vi "KundtsTube2-week7J&J.vi"() -> ()   [LabVIEW 2015]
uses:
  <vilib>/Analysis/NI_AALPro.lvlib
  <vilib>/Analysis/2dsp.llb/Real FFT.vi
  <vilib>/express/express analysis/Spectral/XNode/ExpressSpectralMeasurementsBlockNode.xnode
  <vilib>/express/express analysis/Spectral/Block/exnSpectralBlock spectral measurements RMS poly.vi
  <vilib>/express/express analysis/Spectral/Block/exnSpectralBlock spectral measurements RMS WFM.vi
panel:
  out "?":cdb[](graph)
  out "FFT Graph":cdb[](graph)
  in  "stop":bool
  in  "Time (s)":dbl
  in  "Rate":dbl
  in  "Averages":dbl
  out "Results":T1
  out "Resonance Curve":cluster{"all rows":dbl[], "Array":dbl[]}[](graph)
  in  "Tab Control":enum32{"Simulation", "Experiment"}(tab)
  in  "Input Parameter":T2
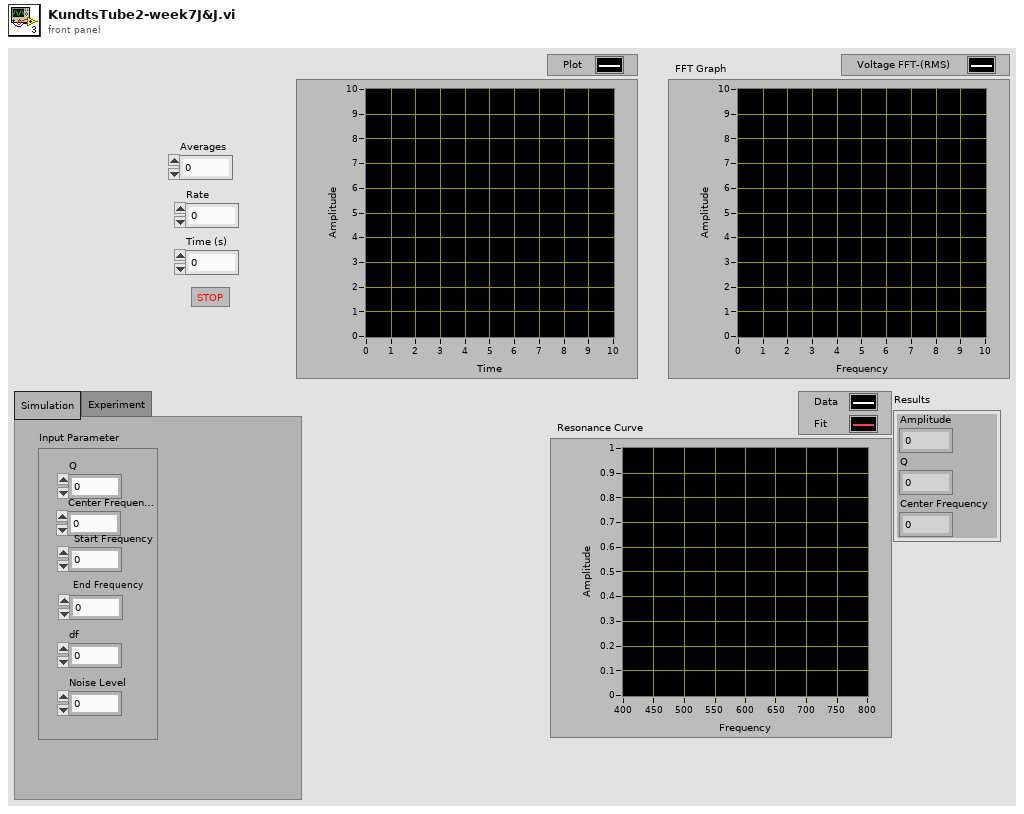
[diagram p1: front panel]
types:
  T1 = cluster{"Amplitude":dbl, "Q":dbl, "Center Frequency":dbl}
  T2 = cluster{"Q":dbl, "Center Frequency":dbl, "Start Frequency":dbl, " End Frequency":dbl, "df":dbl, "Noise Level":dbl}
  T3 = enum16{"open", "replace", "create", "open or create", "replace or create", "replace or create with confirmation"}
  T4 = cluster{"Resonance Curve[0]":cluster{"all rows":dbl[], "Array":dbl[]}, "Resonance Curve[1]":cluster{"all rows":dbl[], "Array":dbl[]}, "Resonance Curve[2]":cluster{"all rows":dbl[], "Array":dbl[]}, "Resonance Curve[3]":cluster{"all rows":dbl[], "Array":dbl[]}, "Resonance Curve[4]":cluster{"all rows":dbl[], "Array":dbl[]}, "Resonance Curve[5]":cluster{"all rows":dbl[], "Array":dbl[]}, "Resonance Curve[6]":cluster{"all rows":dbl[], "Array":dbl[]}, "Resonance Curve[7]":cluster{"all rows":dbl[], "Array":dbl[]}, "Resonance Curve[8]":cluster{"all rows":dbl[], "Array":dbl[]}}
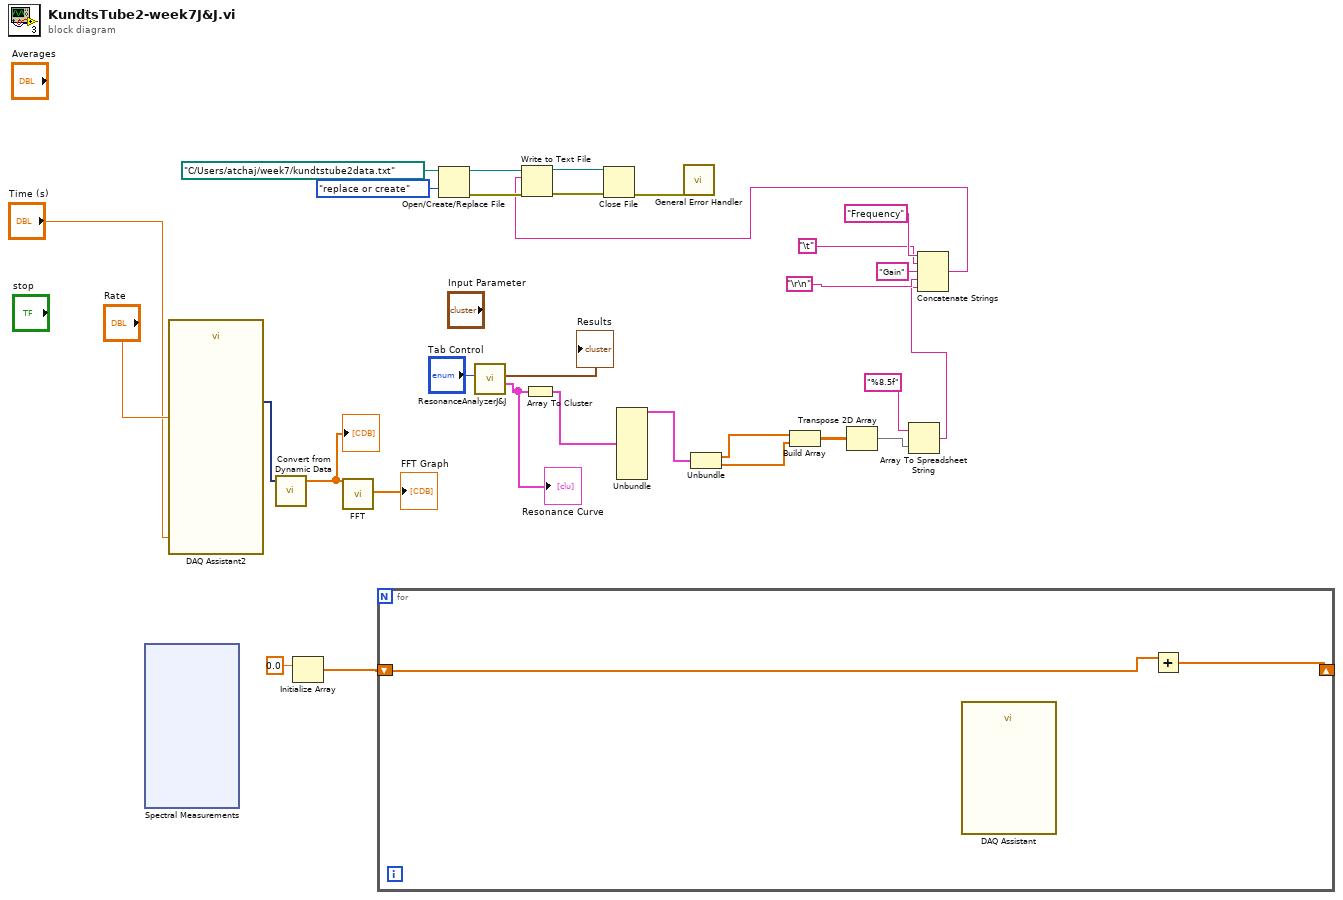
[diagram p0: block diagram]
diagram:
  n1 = xnode "Spectral Measurements"() -> ()  [unwired: 2 in, 3 out]
  n2 = call "DAQ Assistant2"("rate"="Rate", "timeout (s)"="Time (s)") -> ("data"=w5:dynamicdata)  [unwired: 15 in, 2 out]
  n3 = call "Convert from Dynamic Data"("Dynamic Data Type"=w5) -> ("Array"=w4:dbl[])  [unwired: 3 in]
  "?" <- w4
  n4 = Initialize Array(0.0 ("element")) -> (w2:dbl[])  [unwired: 1 in]
  n5 = call-poly <vilib>:"FFT.vi"("X"=w4) -> ("FFT {X}"=→"FFT Graph":cdb[])  [unwired: 9 in, 1 out]
  n6 = for {
    shift-right: [w31] -> _
    shift-left: w2 -> [w32]
    n7 = call "DAQ Assistant"() -> ()  [unwired: 18 in, 2 out]
    n8 = Add(x=w32) -> (x+y=w31:dbl[])  [unwired: 1 in]
  }
  n9 = Open/Create/Replace File(file path (use dialog)=path "C:/Users/atchaj/week7/kundtstube2data.txt", operation (0:open)=T3."replace or create") -> (refnum out=w24:refnum<file>, error out=w25:errorcluster)  [unwired: 4 in, 1 out]
  n10 = call "ResonanceAnalyzerJ&J.vi"("Tab Control"="Tab Control") -> ("Resonance Curve"=w14:cluster{"all rows":dbl[], "Array":dbl[]}[], "Results"=→"Results":T1)  [unwired: 9 in]
  "Resonance Curve" <- w14
  n11 = Array To Cluster(array=w14) -> (cluster=w13:T4)
  n12 = Unbundle(w13) -> ("Resonance Curve[0]"=w12:cluster{"all rows":dbl[], "Array":dbl[]})  [unwired: 8 out]
  n13 = Unbundle(w12) -> ("all rows"=w11:dbl[], "Array"=w10:dbl[])
  n14 = Build Array(w11, w10) -> (w9:dbl[][])
  n15 = Transpose 2D Array(2D array=w9) -> (transposed array=w8:dbl[][])
  n16 = Array To Spreadsheet String(array=w8, 3:"%8.5f" ("format string")) -> (spreadsheet string=w16:string)  [unwired: 1 in]
  n17 = Concatenate Strings("Frequency" ("string"), "\t", "Gain" ("string"), "\r\n", w16) -> (w15:string)
  n18 = Write to Text File(file (use dialog)=w24, text=w15, error in=w25) -> (refnum out=w23:refnum<file>, error out=w26:errorcluster)  [unwired: 1 in, 1 out]
  n19 = Close File(refnum=w23, error in=w26) -> (error out=w27:errorcluster)  [unwired: 1 out]
  n20 = call <vilib>:"General Error Handler.vi"("error in (no error)"=w27) -> ()  [unwired: 10 in, 5 out]
